vi "Settings Dialog.vi"(8 "error in (no error)":errorcluster, 11 "Configuration in":T1={"Hardware Configuration"={"Signal Channel"="PXI1Slot7/ao0", "Response Channel"="PXI1Slot7/ai0", "Trigger Channel"="/PXI1Slot7/PFI0", "Number of Acquisitions"=1.0}, "Analysis Configuration"={"Statistics"=TRUE}, "Signal Type"=enum."From Excel", "New Data Behavior"=enum."Replace", "Signal Configuration"={"Chirp Amplitude"=0.0, "I/O Limit"=0.0, "Sample Rate"=0.0, "Chirp Duration (s)"=0.0, "Upper Frequency"=0.0, "Lower Frequency"=0.0, "Windowing"=enum."None"}, "Waveform File"="", "Save Location"=""}) -> (0 "error out":errorcluster, 2 "UI Refresh Needed?":bool, 3 "Configuration Out":T1={"Hardware Configuration"={"Signal Channel"="PXI1Slot7/ao0", "Response Channel"="PXI1Slot7/ai0", "Trigger Channel"="/PXI1Slot7/PFI0", "Number of Acquisitions"=1.0}, "Analysis Configuration"={"Statistics"=TRUE}, "Signal Type"=enum."From Excel", "New Data Behavior"=enum."Replace", "Signal Configuration"={"Chirp Amplitude"=0.0, "I/O Limit"=0.0, "Sample Rate"=0.0, "Chirp Duration (s)"=0.0, "Upper Frequency"=0.0, "Lower Frequency"=0.0, "Windowing"=enum."None"}, "Waveform File"="", "Save Location"=""})   [LabVIEW 2017]
doc: "Dialog for selecting user specified settings."
uses:
  controls/User Specified Data.ctl
  controls/HW Configuration.ctl
  controls/Analysis Configuration.ctl
  controls/New Data Behavior.ctl
  controls/Signal Configuration.ctl
panel:
  in  "Number of Acquisitions":dbl
  in  "Chirp Windowing":u16(ring) items=["None", "Exponential", "Flat top", "Hamming", "Hanning", "Kaiser-Bessel", "Rectangular"]
  in  "Signal Type":u16(ring) items=["From Excel", "Single Chirp"]
  in  "Chirp Duration (s)":dbl
  in  "Sample Rate (S/s)":dbl
  in  "Lower Freq. (Hz)":dbl
  in  "Upper Freq. (Hz)":dbl
  in  "Input Voltage Limit (V)":dbl
  in  "Chirp Amplitude (V)":dbl
  in  "Trigger Channel":tag="/PXI1Slot7/PFI1"
  in  "Response Channel":tag="PXI1Slot7/ai0"
  in  "Signal Channel":tag="PXI1Slot7/ao0"
  in  "New Data Behavior":u16(ring) items=["Replace", "Overlay", "Append"]
  in  "Cancel Button":bool
  in  "OK Button":bool
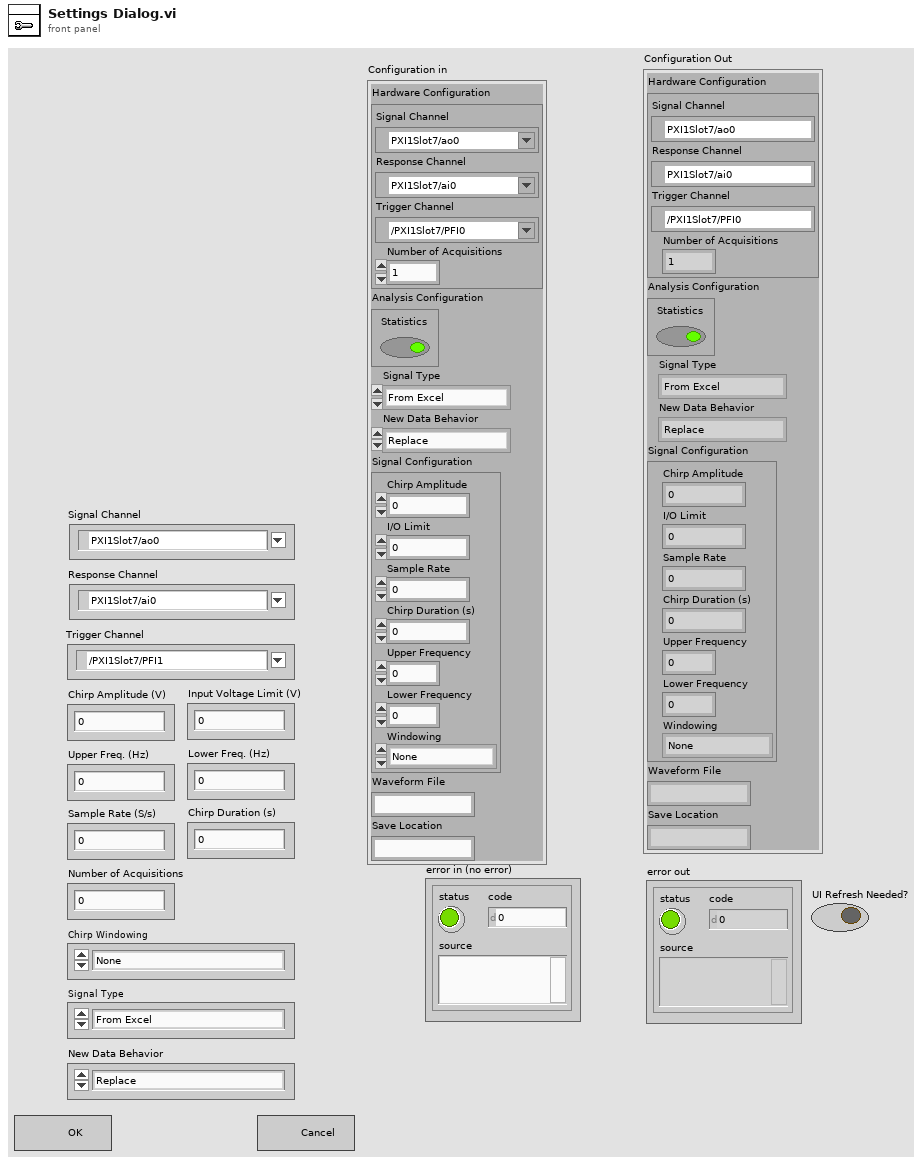
[diagram p1: front panel]
types:
  T1 = typedef "User Specified Data.ctl" = cluster{"Hardware Configuration":T2, "Analysis Configuration":T3, "Signal Type":enum16{"From Excel", "Single Chirp"}, "New Data Behavior":T4, "Signal Configuration":T5, "Waveform File":string, "Save Location":string}
  T2 = typedef "HW Configuration.ctl" = cluster{"Signal Channel":tag, "Response Channel":tag, "Trigger Channel":tag, "Number of Acquisitions":dbl}
  T3 = typedef "Analysis Configuration.ctl" = cluster{"Statistics":bool}
  T4 = typedef "New Data Behavior.ctl" = enum16{"Replace", "Overlay", "Append"}
  T5 = typedef "Signal Configuration.ctl" = cluster{"Chirp Amplitude":dbl, "I/O Limit":dbl, "Sample Rate":dbl, "Chirp Duration (s)":dbl, "Upper Frequency":dbl, "Lower Frequency":dbl, "Windowing":enum16{"None", "Exponential", "Flat top", "Hamming", "Hanning", "Kaiser-Bessel", "Rectangular"}}
  T6 = enum16{"None", "Exponential", "Flat top", "Hamming", "Hanning", "Kaiser-Bessel", "Rectangular"}
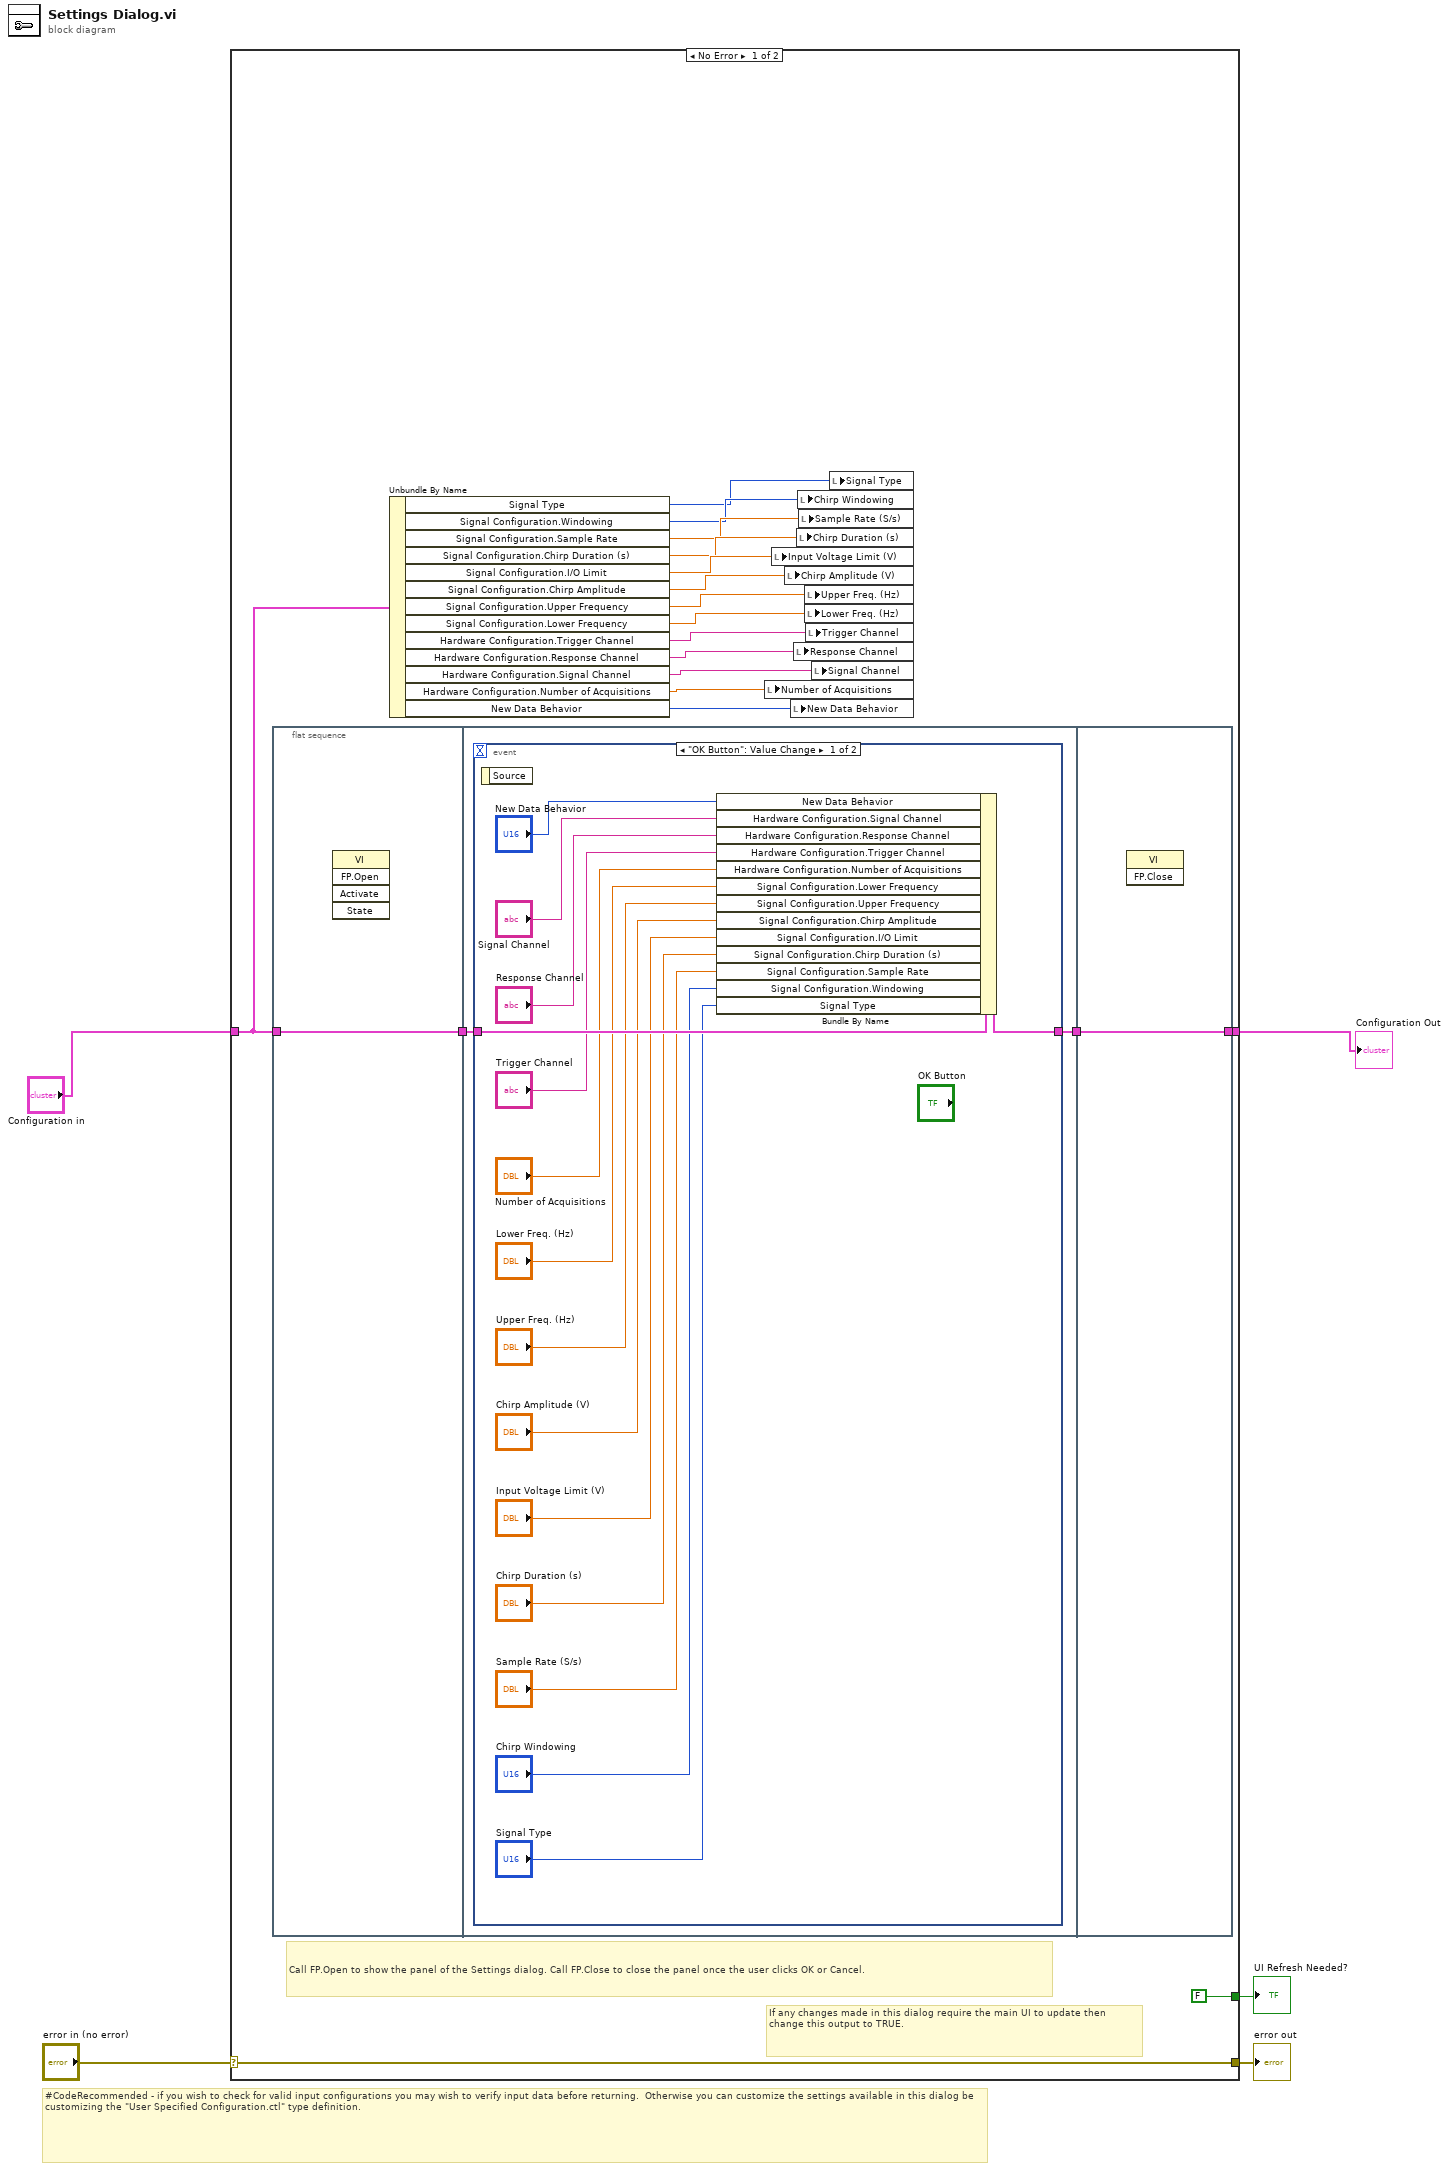
[diagram p0: block diagram]
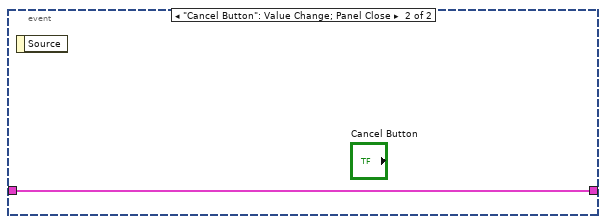
[diagram p2: hidden frame]
diagram:
  # "#CodeRecommended - if you wish to check for valid input configurations you may wish to verify input data before returning.  Otherwise you can customize the settings available in this dialog be customizing the \"User Specified Configuration.ctl\" type definition."
  n1 = case shown="No Error" "error in (no error)" {
    selector: "error in (no error)" -> [w24 w46]
    tunnel: [w24 w46] -> w4
    tunnel: "Configuration in" -> [w21 w45]
    tunnel: [w23 w45] -> w1
    tunnel: [FALSE ("UI Refresh Needed?") _] -> w3
    frame No Error {
      # "Call FP.Open to show the panel of the Settings dialog. Call FP.Close to close the panel once the user clicks OK or Cancel."
      # "If any changes made in this dialog require the main UI to update then change this output to TRUE."
      n2 = flat-sequence {
        tunnel: w21 -> [w25]
        tunnel: [w25] -> w19
        tunnel: w19 -> [w26]
        tunnel: [w27] -> w18
        tunnel: [w44] -> w23
        tunnel: w18 -> [w44]
        frame #0 {
          n3 = invoke class="VI" method="FP.Open"() -> ()  [unwired: 5 in, 5 out]
        }
        frame #1 {
          n4 = event shown="[0] \"OK Button\": Value Change" {
            selector: _ -> [_ _]
            dyn-events: _ -> [_ _]
            timeout: _ -> [_ _]
            tunnel: [w41 w43] -> w27
            tunnel: w26 -> [w42 w43]
            event "OK Button": Value Change {
              n5 = event-data() -> ()  [unwired: 1 in, 1 out]
              n6 = Bundle By Name(cluster=w42, "New Data Behavior"="New Data Behavior", "Hardware Configuration.Signal Channel"="Signal Channel", "Hardware Configuration.Response Channel"="Response Channel", "Hardware Configuration.Trigger Channel"="Trigger Channel", "Hardware Configuration.Number of Acquisitions"="Number of Acquisitions", "Signal Configuration.Lower Frequency"="Lower Freq. (Hz)", "Signal Configuration.Upper Frequency"="Upper Freq. (Hz)", "Signal Configuration.Chirp Amplitude"="Chirp Amplitude (V)", "Signal Configuration.I/O Limit"="Input Voltage Limit (V)", "Signal Configuration.Chirp Duration (s)"="Chirp Duration (s)", "Signal Configuration.Sample Rate"="Sample Rate (S/s)", "Signal Configuration.Windowing"="Chirp Windowing", "Signal Type"="Signal Type") -> (w41:T1)
            }
            event "Cancel Button": Value Change; Panel Close {
              n7 = event-data() -> ()  [unwired: 1 in, 1 out]
            }
          }
        }
        frame #2 {
          n8 = invoke class="VI" method="FP.Close"() -> ()  [unwired: 3 in, 3 out]
        }
      }
      n9 = Unbundle By Name(w21) -> ("Signal Type"=w7:enum16{"From Excel", "Single Chirp"}, "Signal Configuration.Windowing"=w8:T6, "Signal Configuration.Sample Rate"=w9:dbl, "Signal Configuration.Chirp Duration (s)"=w10:dbl, "Signal Configuration.I/O Limit"=w11:dbl, "Signal Configuration.Chirp Amplitude"=w12:dbl, "Signal Configuration.Upper Frequency"=w13:dbl, "Signal Configuration.Lower Frequency"=w14:dbl, "Hardware Configuration.Trigger Channel"=w15:tag, "Hardware Configuration.Response Channel"=w16:tag, "Hardware Configuration.Signal Channel"=w17:tag, "Hardware Configuration.Number of Acquisitions"=w6:dbl, "New Data Behavior"=w20:T4)
      n10 = local write "Number of Acquisitions"(w6) -> ()
      n11 = local write "Input Voltage Limit (V)"(w11) -> ()
      n12 = local write "Chirp Amplitude (V)"(w12) -> ()
      n13 = local write "New Data Behavior"(w20) -> ()
      n14 = local write "Response Channel"(w16) -> ()
      n15 = local write "Chirp Duration (s)"(w10) -> ()
      n16 = local write "Chirp Windowing"(w8) -> ()
      n17 = local write "Sample Rate (S/s)"(w9) -> ()
      n18 = local write "Upper Freq. (Hz)"(w13) -> ()
      n19 = local write "Lower Freq. (Hz)"(w14) -> ()
      n20 = local write "Trigger Channel"(w15) -> ()
      n21 = local write "Signal Channel"(w17) -> ()
      n22 = local write "Signal Type"(w7) -> ()
    }
    frame Error {
    }
  }
  "UI Refresh Needed?" <- w3
  "error out" <- w4
  "Configuration Out" <- w1
